vi "Dialog Window Setup_Pre-Populate.vi"(7 "Action":enum16{"Pre-Populate", "Post-Populate"}(ring), 8 "error in":errorcluster, 10 "Dialog VI Ref In [Parent]":refnum<vi>, 11 "Scripted VI Ref":refnum<vi>) -> (0 "error out":errorcluster, 2 "Dialog VI Ref Out":refnum<vi>)   [LabVIEW 2023]
doc: "Align Dialog to scripted block diagram window, prepare dialog FP (resizing) and open it for view. If Dialog ref is not passesd in it's assumed to be the parent of this VI."
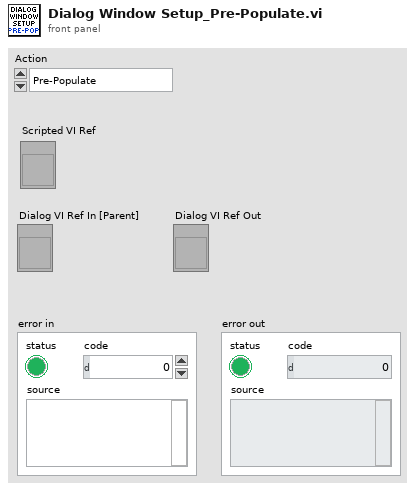
[diagram p1: front panel]
types:
  T1 = enum32{"Invalid", "Standard", "Closed", "Hidden", "Minimized", "Maximized"}
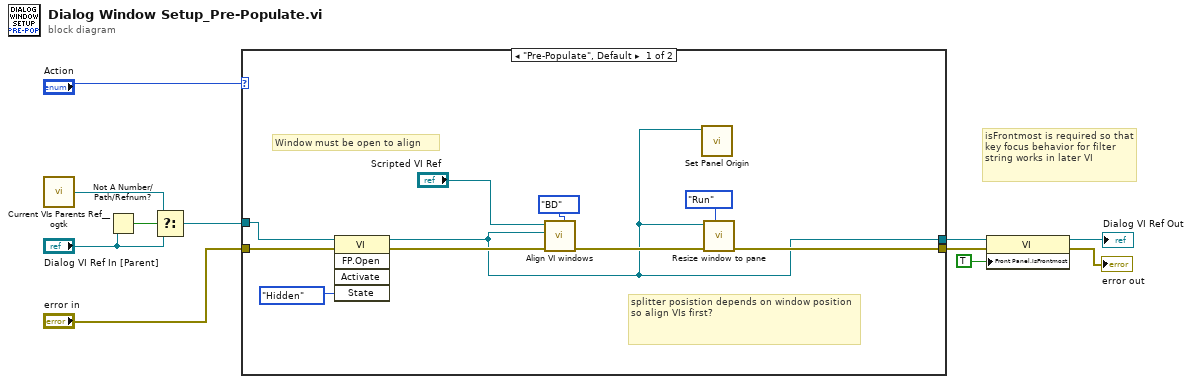
[diagram p0: block diagram]
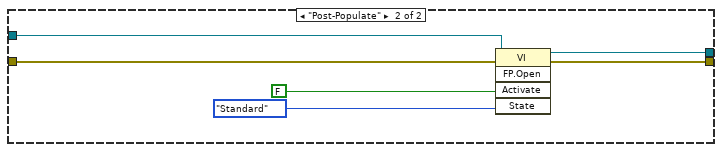
[diagram p2: hidden frame]
diagram:
  # "isFrontmost is required so that key focus behavior for filter string works in later VI"
  n1 = call <userlib>:"Current VIs Parents Ref__ogtk.vi"() -> ("Calling VI's Reference"=w10:refnum<vi>)  [unwired: 2 in]
  n2 = Not A Number/Path/Refnum?(number/path/refnum="Dialog VI Ref In [Parent]") -> (NaN/Path/Refnum?=w7:bool)
  n3 = Select(t=w10, s=w7, f="Dialog VI Ref In [Parent]") -> (s? t:f=w9:refnum<vi>)
  n4 = case shown="\"Pre-Populate\", Default" "Action" {
    tunnel: [w12 w25] -> w3
    tunnel: [w16 w27] -> w5
    tunnel: w9 -> [w20 w22]
    tunnel: "error in" -> [w19 w23]
    frame "Pre-Populate", Default {
      # "splitter posistion depends on window position so align VIs first?"
      # "Window must be open to align"
      n5 = invoke class="VI" method="FP.Open"(reference=w20, error in=w19, "State"=T1."Hidden") -> (reference out=w12:refnum<vi>, error out=w15:errorcluster)  [unwired: 2 in, 3 out]
      n6 = call "Align VI windows.vi"("Align to"=enum16{"FP", "BD"}."BD", "error in"=w15, "VI to Move Ref"=w12, "Stationary VI Ref"="Scripted VI Ref") -> ("error out"=w17:errorcluster)  [unwired: 7 in]
      n7 = call "Set Panel Origin.vi"("VI Ref In"=w12) -> ()  [unwired: 9 in, 2 out]
      n8 = call "Resize window to pane.vi"("Mode"=enum16{"Run", "Development"}."Run", "error in"=w17, "VI Ref In"=w12) -> ("error out"=w16:errorcluster)  [unwired: 7 in, 1 out]
    }
    frame "Post-Populate" {
      n9 = invoke class="VI" method="FP.Open"(reference=w22, error in=w23, "Activate"=FALSE ("Activate?"), "State"=T1."Standard") -> (reference out=w25:refnum<vi>, error out=w27:errorcluster)  [unwired: 1 in, 3 out]
    }
  }
  n10 = property class="VI"(reference=w3, error in=w5, "Front Panel.IsFrontmost"=TRUE ("Front Panel Window:Is Frontmost")) -> (reference out=→"Dialog VI Ref Out":refnum<vi>, error out=→"error out":errorcluster)
